vi "InitTestFilePath.vi"(8 "ErrorArray In":errorcluster[](array[cluster]), 10 "clFrontPanelControlRefs In":T1) -> (0 "ErrorArray Out":errorcluster[](array[cluster]), 2 "clFrontPanelControlRefs Out":T1)   [LabVIEW 2014]
uses:
  <vilib>/Utility/config.llb/NI_LVConfig.lvlib
  <userlib>/NIST/NISTErrorLib/NISTErrorLib.lvlib
  Config_class/Config.lvclass
  <vilib>/Utility/config.llb/Read Key (Path).vi
  FrontPanel/TypeDefs/clFrontPanelControlRefs.ctl
  Framework.lvlib
  FrontPanel/TypeDefs/clEventConfig.ctl
  Modules/PmuImpairPlugins/PmuImpairPluginBase_class/TypeDefs/clImpairConfig.ctl
  Modules/PmuImpairPlugins/PmuImpairPluginBase_class/PmuImpairPluginBase.lvclass
panel:
  # "When you add a control \non the front panel, add a\nreference for it in this\ntype def.  This cluster\nwill hold all of the refer-\nences to the front panel\ncontrols in order to pass\nthese control references \nto subvis."
  # "When you add a control \non the front panel, add a\nreference for it in this\ntype def.  This cluster\nwill hold all of the refer-\nences to the front panel\ncontrols in order to pass\nthese control references \nto subvis."
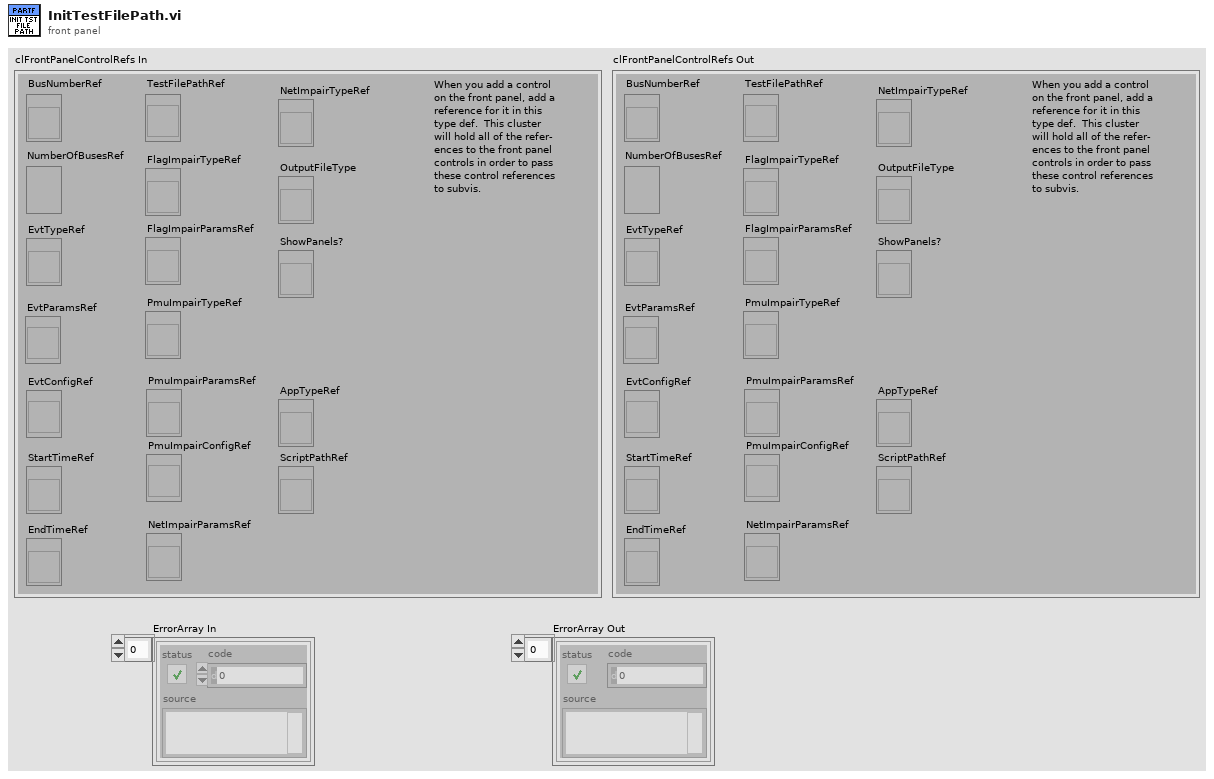
[diagram p1: front panel]
types:
  T1 = typedef "Framework.lvlib/clFrontPanelControlRefs.ctl" = cluster{"TestFilePathRef":refnum<vi>, "BusNumberRef":refnum<vi>, "NumberOfBusesRef":refnum<vi>, "EvtTypeRef":refnum<vi>, "EvtParamsRef":refnum<vi>, "EvtConfigRef":refnum<vi>, "StartTimeRef":refnum<vi>, "EndTimeRef":refnum<vi>, "PmuImpairTypeRef":refnum<vi>, "PmuImpairParamsRef":refnum<vi>, "NetImpairParamsRef":refnum<vi>, "FlagImpairTypeRef":refnum<vi>, "FlagImpairParamsRef":refnum<vi>, "NetImpairTypeRef":refnum<vi>, "OutputFileType":refnum<vi>, "PmuImpairConfigRef":refnum<vi>, "AppTypeRef":refnum<vi>, "ScriptPathRef":refnum<vi>, "ShowPanels?":refnum<vi>}
  T2 = typedef "Framework.lvlib/Config.lvclass/RootDir.ctl" = cluster{"pathRootDir":path, "btnOutPath":bool, "OutDir":string, "btnOpenOutputDir":bool, "ScriptDir":string, "btnOpenScriptDir":bool, "TestDir":string, "btnOpenTestDir":bool}
  T3 = typedef "NI_LVConfig.lvlib/Config Data RefNum.ctl" = refnum<k1>
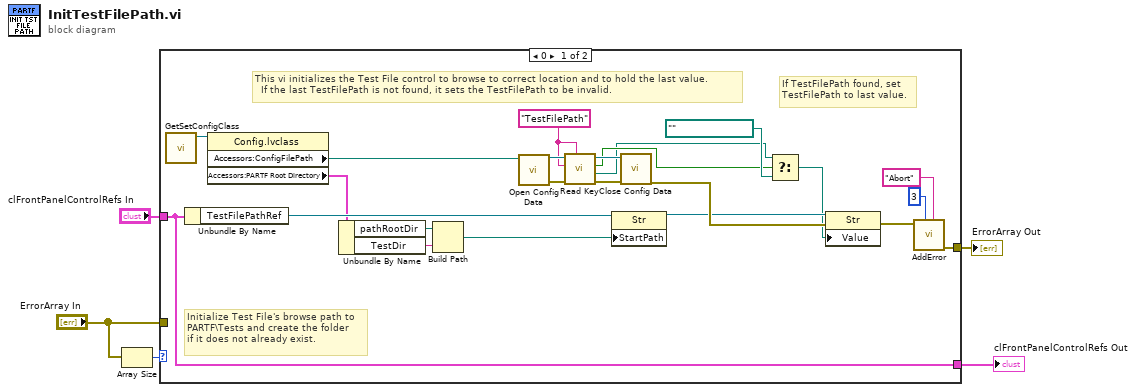
[diagram p0: block diagram]
diagram:
  n1 = Array Size(array="ErrorArray In") -> (size(s)=w4:i32)
  n2 = case shown="0" w4 {
    tunnel: [w24 w30] -> w5
    tunnel: "ErrorArray In" -> [_ w30]
    tunnel: "clFrontPanelControlRefs In" -> [w19 w29]
    tunnel: [w19 w29] -> w1
    frame 0 {
      w18 = "TestFilePath" ("key")
      # "If TestFilePath found, set\nTestFilePath to last value."
      # "Initialize Test File's browse path to\nPARTF\\Tests and create the folder\nif it does not already exist."
      # "This vi initializes the Test File control to browse to correct location and to hold the last value.\n  If the last TestFilePath is not found, it sets the TestFilePath to be invalid."
      n3 = call "GetSetConfigClass.vi"() -> ("Ref out"=w23:refnum<class "Config.lvclass">)  [unwired: 11 in]
      n4 = Unbundle By Name(w19) -> ("TestFilePathRef"=w17:refnum<vi>)
      n5 = property class="Config.lvclass"(reference=w23) -> ("Accessors:ConfigFilePath"=w22:path, "Accessors:PARTF Root Directory"=w13:T2)  [unwired: 1 in, 2 out]
      n6 = Unbundle By Name(w13) -> ("pathRootDir"=w12:path, "TestDir"=w11:string)
      n7 = Build Path(base path=w12, name or relative path=w11) -> (appended path=w10:path)
      n8 = call <vilib>:"Open Config Data.vi"("configuration file path"=w22) -> ("error out"=w28:errorcluster, "refnum"=w27:T3)  [unwired: 8 in, 1 out]
      n9 = call-poly <vilib>:"Read Key.vi"("section"=w18, "error in (no error)"=w28, "key"=w18, "refnum"=w27) -> ("error out"=w26:errorcluster, "value"=w6:path, "found?"=w8:bool, "refnum out"=w25:T3)  [unwired: 4 in]
      n10 = property class="Str"(reference=w17, "StartPath"=w10) -> (reference out=w15:refnum<vi>)  [unwired: 1 in, 1 out]
      n11 = call <vilib>:"Close Config Data.vi"("error in (no error)"=w26, "refnum"=w25) -> ("error out"=w16:errorcluster)  [unwired: 8 in, 1 out]
      n12 = Select(t=w6, s=w8, f=path "" ("Blank Path")) -> (s? t:f=w7:path)
      n13 = property class="Str"(reference=w15, error in=w16, "Value"=w7) -> (error out=w14:errorcluster)  [unwired: 1 out]
      n14 = call <userlib>:"AddError.vi"("Severity"="Abort" ("String"), "Priority"=u8 3, "error in (no error)"=w14) -> ("ErrorArray"=w24:errorcluster[])  [unwired: 7 in, 1 out]
    }
    frame 1, Default {
    }
  }
  "ErrorArray Out" <- w5
  "clFrontPanelControlRefs Out" <- w1
